vi "Word_Open.vi"(0 "word application in":refnum<k7>, 5 "window state":T1(ring), 7 "display alerts?":bool=TRUE, 11 "Error in":errorcluster) -> (4 "word application out":refnum<k7>, 8 "application already open":bool, 10 "version":string, 15 "Error out":errorcluster)   [LabVIEW 2020, in "NI_ReportGenerationToolkit.lvlib"]
uses:
  <vilib>/addons/_office/NI_ReportGenerationToolkit.lvlib
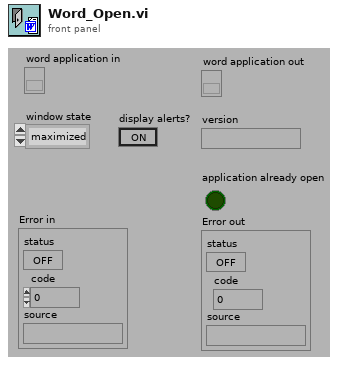
[diagram p1: front panel]
types:
  T1 = enum16{"maximized", "minimized", "normal", "no change"}
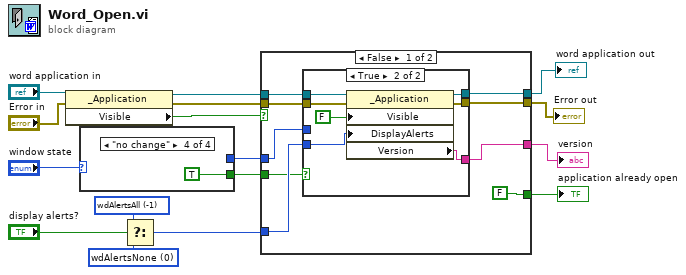
[diagram p0: block diagram]
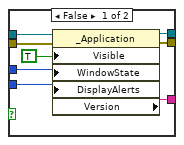
[diagram p2: hidden frame]
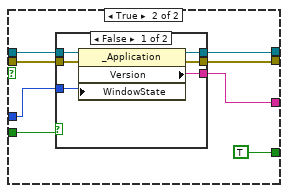
[diagram p3: hidden frame]
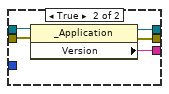
[diagram p4: hidden frame]
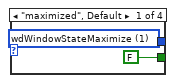
[diagram p5: hidden frame]
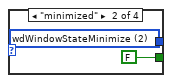
[diagram p6: hidden frame]
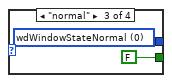
[diagram p7: hidden frame]
diagram:
  w13 = -1 items=["wdAlertsNone"=0, "wdAlertsMessageBox"=-2, "wdAlertsAll"=-1] ("DisplayAlerts")
  w12 = 0 items=["wdAlertsNone"=0, "wdAlertsMessageBox"=-2, "wdAlertsAll"=-1] ("DisplayAlerts")
  n1 = property class="_Application"(reference="word application in", error in="Error in") -> (reference out=w5:refnum<k7>, error out=w4:errorcluster, "Visible"=w3:bool)
  n2 = case shown="\"no change\"" "window state" {
    tunnel: [w18 w20 w22 _] -> w9
    tunnel: [FALSE FALSE FALSE TRUE] -> w1
    frame "maximized", Default {
      w18 = 1 items=["wdWindowStateNormal", "wdWindowStateMaximize", "wdWindowStateMinimize"] ("WindowState")
    }
    frame "minimized" {
      w20 = 2 items=["wdWindowStateNormal", "wdWindowStateMaximize", "wdWindowStateMinimize"] ("WindowState")
    }
    frame "normal" {
      w22 = 0 items=["wdWindowStateNormal", "wdWindowStateMaximize", "wdWindowStateMinimize"] ("WindowState")
    }
    frame "no change" {
    }
  }
  n3 = Select(t=w13, s="display alerts?", f=w12) -> (s? t:f=w11:i32)
  n4 = case shown="False" w3 {
    tunnel: [w32 w50] -> w16
    tunnel: [w31 w52] -> w15
    tunnel: w11 -> [w27 _]
    tunnel: w9 -> [w26 w53]
    tunnel: [w30 w51] -> w8
    tunnel: w5 -> [w29 w55]
    tunnel: w4 -> [w28 w54]
    tunnel: [FALSE TRUE] -> w2
    tunnel: w1 -> [w24 w48]
    frame False {
      n5 = case shown="True" w24 {
        tunnel: [w40 w42] -> w32
        tunnel: [w39 w45] -> w31
        tunnel: [w38 w41] -> w30
        tunnel: w29 -> [w37 w44]
        tunnel: w28 -> [w36 w43]
        tunnel: w27 -> [w35 w46]
        tunnel: w26 -> [w34 _]
        frame False {
          n6 = property class="_Application"(reference=w37, error in=w36, "Visible"=TRUE, "WindowState"=w34, "DisplayAlerts"=w35) -> (reference out=w40:refnum<k7>, error out=w38:errorcluster, "Version"=w39:string)
        }
        frame True {
          n7 = property class="_Application"(reference=w44, error in=w43, "Visible"=FALSE, "DisplayAlerts"=w46) -> (reference out=w42:refnum<k7>, error out=w41:errorcluster, "Version"=w45:string)
        }
      }
    }
    frame True {
      n8 = case shown="False" w48 {
        tunnel: w55 -> [w61 w66]
        tunnel: w54 -> [w60 w62]
        tunnel: w53 -> [w59 _]
        tunnel: [w58 w63] -> w52
        tunnel: [w57 w64] -> w51
        tunnel: [w56 w65] -> w50
        frame False {
          n9 = property class="_Application"(reference=w61, error in=w60, "WindowState"=w59) -> (reference out=w56:refnum<k7>, error out=w57:errorcluster, "Version"=w58:string)
        }
        frame True {
          n10 = property class="_Application"(reference=w66, error in=w62) -> (reference out=w65:refnum<k7>, error out=w64:errorcluster, "Version"=w63:string)
        }
      }
    }
  }
  "word application out" <- w16
  "Error out" <- w8
  "version" <- w15
  "application already open" <- w2
